vi "get_user.vi"(8 "error in (no error)":errorcluster) -> (0 "error out":errorcluster, 2 "username out":string)   [LabVIEW 2010, in "XUserDropdown.xctl"]
uses:
  XUserDropdown/global_variable.vi
  XUserDropdown/XUserDropdown.xctl
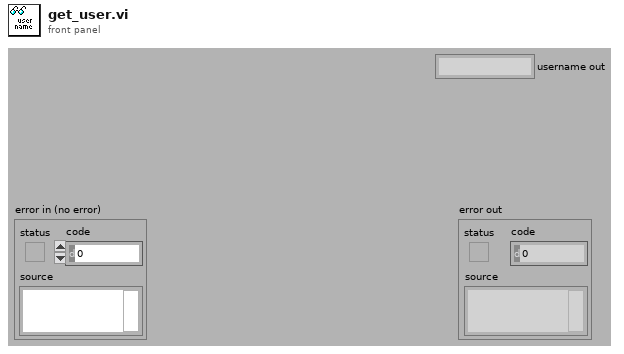
[diagram p1: front panel]
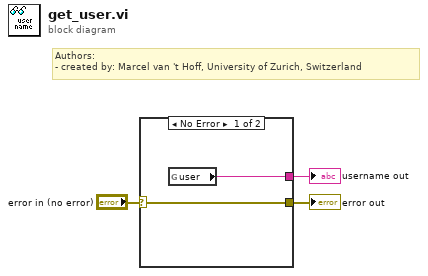
[diagram p0: block diagram]
diagram:
  # "Authors: \n- created by: Marcel van 't Hoff, University of Zurich, Switzerland"
  n1 = case shown="No Error" "error in (no error)" {
    selector: "error in (no error)" -> [w5 w6]
    tunnel: [w5 w6] -> w2
    tunnel: [w4 _] -> w1
    frame No Error {
      n2 = global read "global_variable.vi" "user"() -> (w4:string)
    }
    frame Error {
    }
  }
  "error out" <- w2
  "username out" <- w1
